vi "Servo.vi"(0 "period (20Mhz)":u32=60606, 1 "(2.5us)":u32, 2 "Servo DIO":refnum<k21>) -> ()   [LabVIEW 2019]
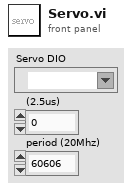
[diagram p1: front panel]
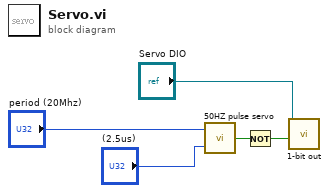
[diagram p0: block diagram]
diagram:
  n1 = call "50HZ pulse servo.vi"("(2.5us)"="(2.5us)", "period (20Mhz)"="period (20Mhz)") -> ("50HZ pulse"=w5:bool)
  n2 = Not(x=w5) -> (.not. x?=w2:bool)
  n3 = call "1-bit out.vi"("OUT"=w2, "DIO Refnum"="Servo DIO") -> ()  [unwired: 10 in]
